vi "Set Text.vi"(8 "error in (no error)":errorcluster, 10 "Text":string, 11 "ScintillaNET in":refnum<class "ScintillaNET.lvclass">) -> (0 "error out":errorcluster, 3 "ScintillaNET out":refnum<class "ScintillaNET.lvclass">)   [LabVIEW 2018, in "ScintillaNET.lvclass"]
uses:
  ScintillaNET.lvclass
  ScintillaNET.lvclass/ScintillaNET.ctl
  D:/project/hobby/LF2R/LabVIEW/source/ScintillaNET/dll/ScintillaNET.dll
  dll/ScintillaNET.dll
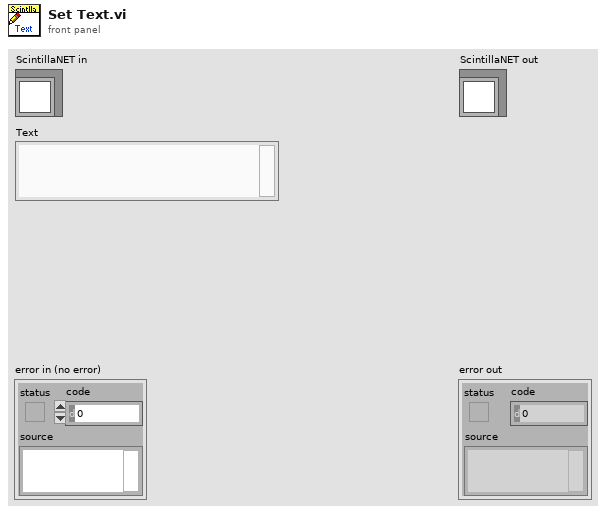
[diagram p1: front panel]
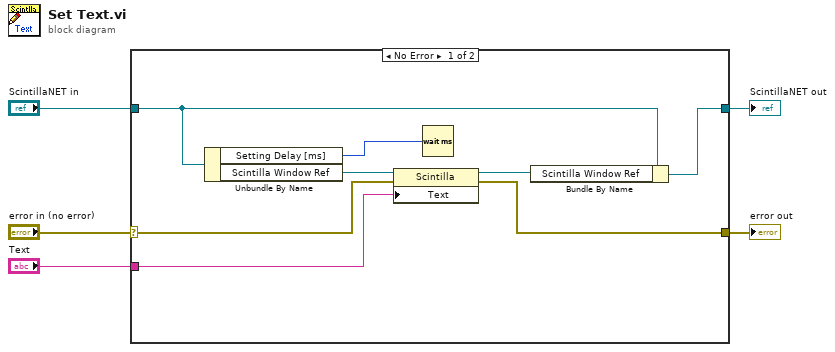
[diagram p0: block diagram]
diagram:
  n1 = case shown="No Error" "error in (no error)" {
    selector: "error in (no error)" -> [w12 w15]
    tunnel: [w11 w15] -> w4
    tunnel: [w13 w14] -> w2
    tunnel: "ScintillaNET in" -> [w9 w14]
    tunnel: "Text" -> [w7 _]
    frame No Error {
      n2 = Unbundle By Name(w9) -> ("Setting Delay [ms]"=w6:u32, "Scintilla Window Ref"=w8:refnum<k24>)
      n3 = property class="Scintilla"(reference=w8, error in=w12, "Text"=w7) -> (reference out=w10:refnum<k24>, error out=w11:errorcluster)
      n4 = Wait (ms)(milliseconds to wait=w6) -> ()  [unwired: 1 out]
      n5 = Bundle By Name(cluster=w9, "Scintilla Window Ref"=w10) -> (w13:refnum<class "ScintillaNET.lvclass">)
    }
    frame Error {
    }
  }
  "error out" <- w4
  "ScintillaNET out" <- w2
